vi "Read ACIR Setting.vi"(8 "error in (no error)":errorcluster, 11 "ACIR configuration":refnum<class "ACIR configuration.lvclass">) -> (0 "error out":errorcluster, 2 "ACIR Setting":T1 {"Frequency" format="%#_6p"}, 3 "ACIR configuration out":refnum<class "ACIR configuration.lvclass">)   [LabVIEW 2025, in "ACIR.lvlib" / "ACIR configuration.lvclass"]
uses:
  ACIR configuration.lvclass
  ACIR Instrument Setting.ctl
  ACIR configuration.lvclass/ACIR configuration.ctl
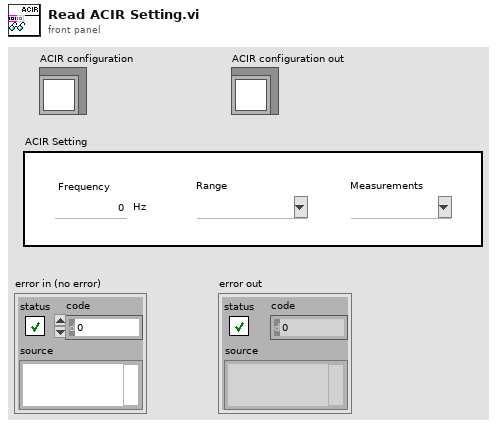
[diagram p1: front panel]
types:
  T1 = typedef "ACIR.lvlib/ACIR configuration.lvclass/ACIR Instrument Setting.ctl" = cluster{"Frequency":dbl, "Range":string, "Measurements":string}
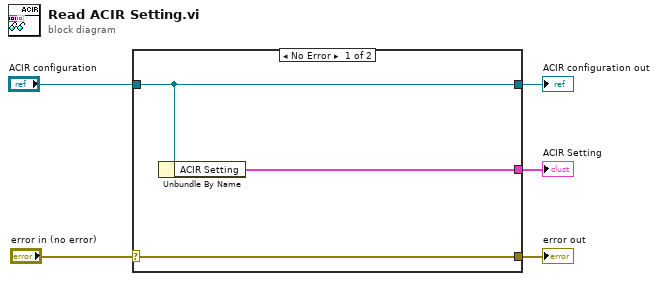
[diagram p0: block diagram]
diagram:
  n1 = case shown="No Error" "error in (no error)" {
    selector: "error in (no error)" -> [w8 w9]
    tunnel: [w8 w9] -> w4
    tunnel: [w7 w10] -> w2
    tunnel: "ACIR configuration" -> [w7 w10]
    tunnel: [w6 _] -> w1
    frame No Error {
      n2 = Unbundle By Name(w7) -> ("ACIR Setting"=w6:T1)
    }
    frame Error {
    }
  }
  "error out" <- w4
  "ACIR configuration out" <- w2
  "ACIR Setting" <- w1
